vi "LinearThrottle.vi"(8 "Maximum":dbl=1.0 format="%#_13g", 9 "Minimum":dbl format="%#_13g", 10 "Throttle":dbl format="%#_13g", 11 "Value":dbl format="%#_13g") -> (3 "Numeric":dbl format="%#_13g")   [LabVIEW 2014]
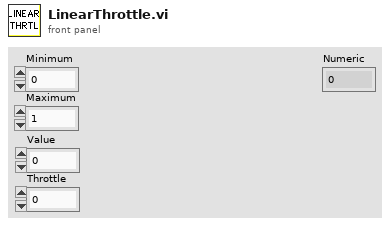
[diagram p1: front panel]
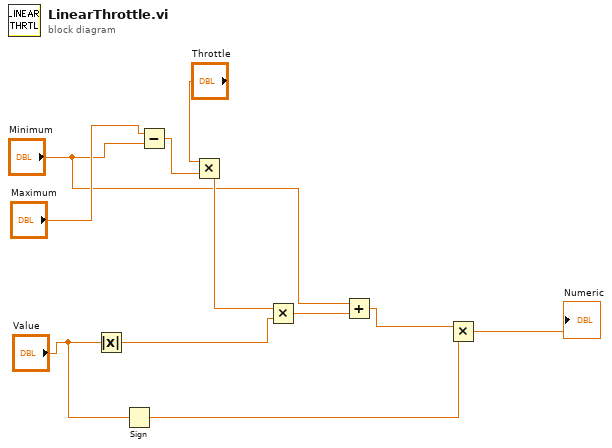
[diagram p0: block diagram]
diagram:
  n1 = Absolute Value(x="Value") -> (abs(x)=w4:dbl)
  n2 = Sign(1:"Value") -> (0:w10:dbl)
  n3 = Subtract(x="Maximum", y="Minimum") -> (x-y=w5:dbl)
  n4 = Multiply(x="Throttle", y=w5) -> (x*y=w7:dbl)
  n5 = Multiply(x=w7, y=w4) -> (x*y=w2:dbl)
  n6 = Add(x="Minimum", y=w2) -> (x+y=w1:dbl)
  n7 = Multiply(x=w1, y=w10) -> (x*y=→"Numeric":dbl)
